vi "Compile UEGO Channels.vi"(8 "error in (no error)":errorcluster, 10 "Name":string, 11 "Device Item Ref in":T6 format="%.0x") -> (0 "error out":errorcluster, 1 "UEGO Engine Data":T2 {"Ordered Channels" format="%.0x"; "RT IDs"."Slot #" max=15; "RT IDs"."Chip Address (A2 A1 A0)" max=7}, 2 "Initial UEGO SPI CMDs":u64[](array[numeric]), 3 "Device Item Ref out":T6 format="%.0x", 5 "RT UEGO Settling Time Data":T1)   [LabVIEW 2014, in "SLSC configuration System Explorer.lvlib"]
uses:
  SLSC configuration System Explorer.lvlib
  <vilib>/NI Veristand/Custom Device API/Custom Device Item Ref.ctl
  Shared/Type Defs/RT Engine Data.ctl
  Shared/Type Defs/RT IDs.ctl
  Shared/SPI Utility/Slot #.ctl
  Shared/MCP23S17/Chip Address.ctl
  Engine/Type Defs/RT UEGO Setting Time Data.ctl
  Shared/UEGO Board/Bank Calibration States.ctl
  Shared/UEGO Board/Calibration State.ctl
  Shared/Constants.vi
  <vilib>/NI Veristand/Custom Device API/Get Item Property (U32).vi
  <vilib>/NI Veristand/Custom Device Tools/Custom Device Utility Library/Custom Device Utility Library.lvlib
  Shared/SLSC configuration Shared.lvlib
  <vilib>/NI Veristand/Custom Device API/Custom Device API.lvlib
  Engine/SLSC configuration Engine.lvlib
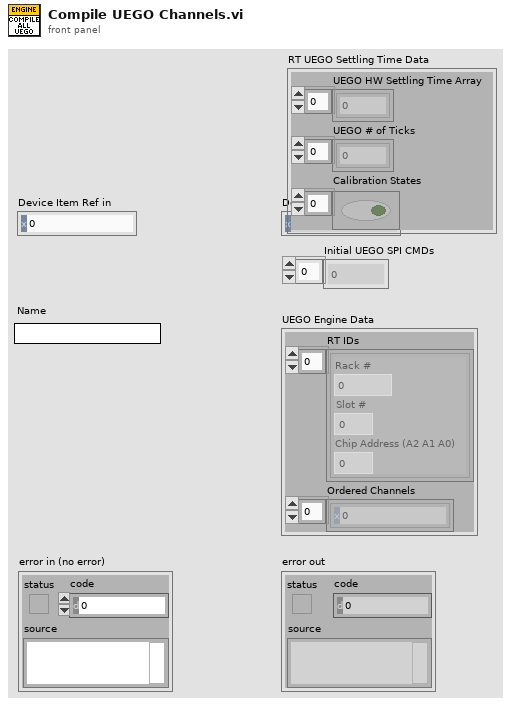
[diagram p1: front panel]
types:
  T1 = typedef "SLSC configuration Engine.lvlib/RT UEGO Setting Time Data.ctl" = cluster{"UEGO HW Settling Time Array":u32[], "UEGO # of Ticks":u32[], "Calibration States":bool[]}
  T2 = typedef "SLSC configuration Shared.lvlib/RT Engine Data.ctl" = cluster{"RT IDs":T3[], "Ordered Channels":T6[]}
  T3 = typedef "SLSC configuration Shared.lvlib/RT IDs.ctl" = cluster{"Rack #":u8, "Slot #":T4, "Chip Address (A2 A1 A0)":T5}
  T4 = typedef "SLSC configuration Shared.lvlib/Slot #.ctl" = u8
  T5 = typedef "SLSC configuration Shared.lvlib/Chip Address.ctl" = u8
  T6 = typedef "Custom Device API.lvlib/Custom Device Item Ref.ctl" = u64
  T7 = typedef "SLSC configuration Shared.lvlib/Bank Calibration States.ctl" = T8[]
  T8 = typedef "SLSC configuration Shared.lvlib/Calibration State.ctl" = bool
  T9 = typedef "SLSC configuration Shared.lvlib/Card Position.ctl" = cluster{"Rack #":u8, "Slot #":T4}
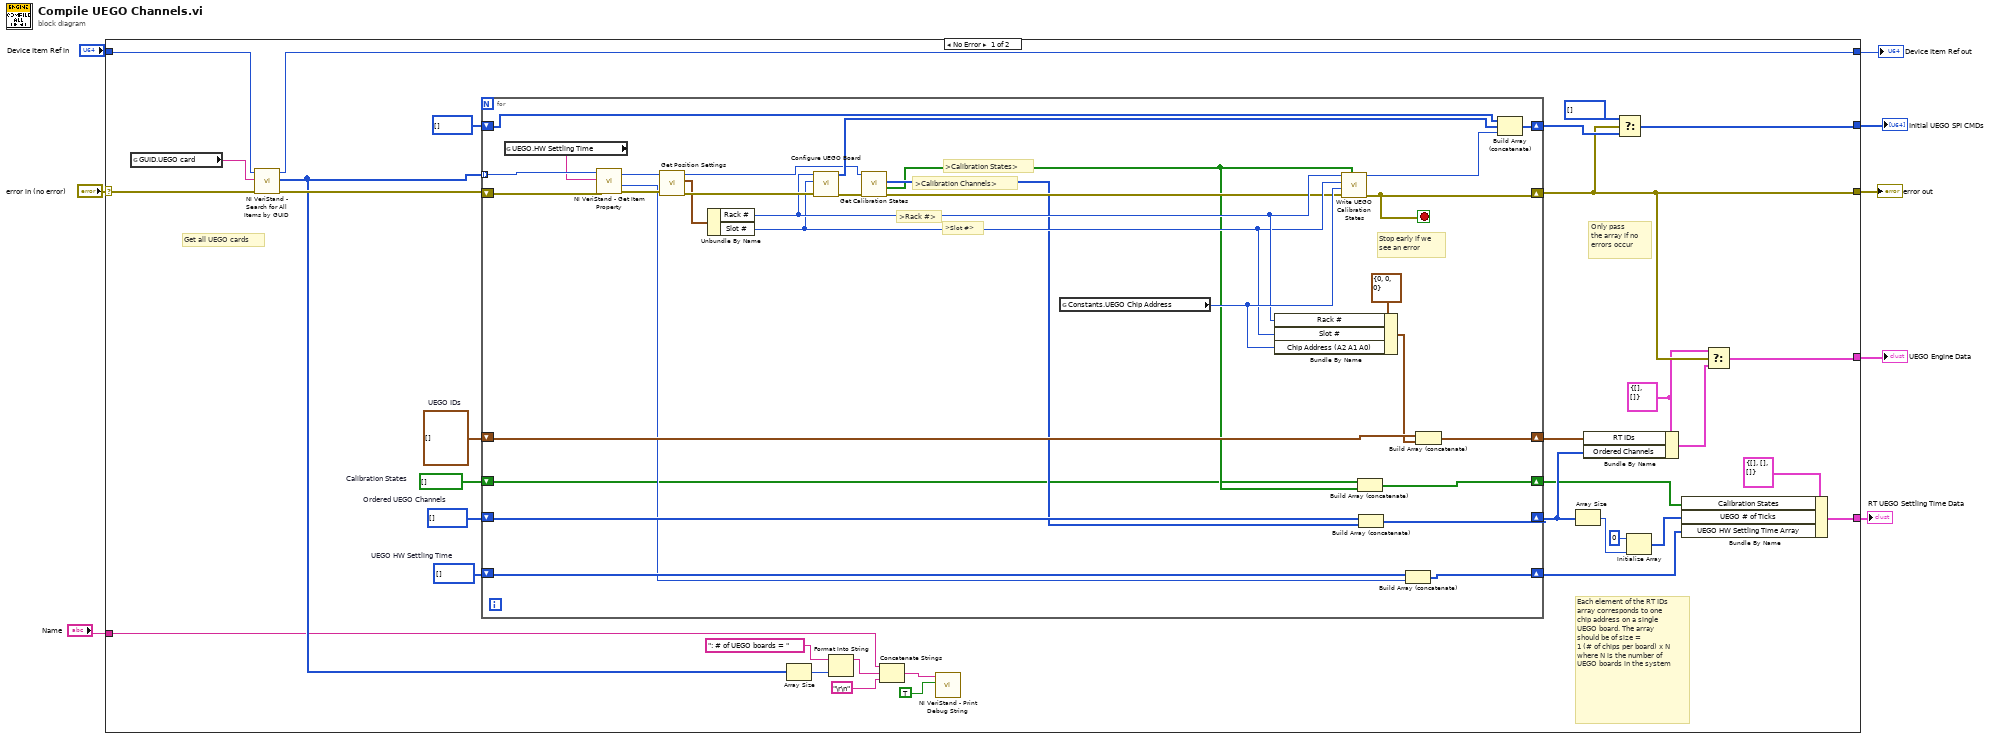
[diagram p0: block diagram]
diagram:
  n1 = case shown="No Error" "error in (no error)" {
    selector: "error in (no error)" -> [w40 w75]
    tunnel: [w30 w75] -> w8
    tunnel: "Device Item Ref in" -> [w35 w74]
    tunnel: [w27 _] -> w5
    tunnel: [w31 _] -> w4
    tunnel: [w34 w74] -> w3
    tunnel: "Name" -> [w19 _]
    tunnel: [w12 _] -> w1
    frame No Error {
      w10 = T7 []  # Calibration States
      w18 = u32[] []  # UEGO HW Settling Time
      w29 = T2 {"RT IDs"=[], "Ordered Channels"=[]} ("FIU Engine Data")
      w37 = T6[] []  # Ordered UEGO Channels
      w38 = T3[] []  # UEGO IDs
      # "Only pass\nthe array if no\nerrors occur"
      # "Get all UEGO cards"
      # "Each element of the RT IDs array corresponds to one chip address on a single UEGO board. The array should be of size =\n1 (# of chips per board) x N where N is the number of UEGO boards in the system"
      n2 = global read "Constants.vi" "GUID.UEGO card"() -> (w42:string)
      n3 = call <vilib>:"NI VeriStand - Search for All Items by GUID.vi"("error in"=w40, "Item GUID"=w42, "Section Ref in"=w35) -> ("error out"=w41:errorcluster, "Item Refs"=w20:T6[], "Section Ref out"=w34:T6)  [unwired: 5 in, 1 out]
      n4 = for {
        tunnel: w20 -> [w53] mode=indexing
        shift-right: [w65] -> w30
        shift-left: w41 -> [w54]
        shift-right: [w70] -> w33
        shift-left: u64[] [] ("SPI FIFO Messages") -> [w73]
        shift-right: [w68] -> w36
        shift-left: w38 -> [w69]
        shift-right: [w66] -> w17
        shift-left: w37 -> [w67]
        shift-right: [w47] -> w13
        shift-left: w18 -> [w48]
        shift-right: [w43] -> w9
        shift-left: w10 -> [w44]
        stop <- w65 stop-if-true
        # ">Calibration States>"
        # "Stop early if we\nsee an error"
        # ">Calibration Channels>"
        # ">Slot #>"
        # ">Rack #>"
        n5 = global read "Constants.vi" "UEGO.HW Settling Time"() -> (w50:string)
        n6 = call-poly <vilib>:"NI VeriStand - Get Item Property.vi"("error in (no error)"=w54, "Property Name"=w50, "Item Ref in"=w53) -> ("error out"=w52:errorcluster, "Value"=w46:u32, "Item Ref out"=w51:T6)  [unwired: 5 in, 1 out]
        n7 = call "Get Position Settings.vi"("error in (no error)"=w52, "Item Ref in"=w51) -> ("error out"=w61:errorcluster, "Card Position"=w60:T9, "Item Ref out"=w56:T6)  [unwired: 7 in]
        n8 = Unbundle By Name(w60) -> ("Rack #"=w59:u8, "Slot #"=w58:T4)
        n9 = call "Configure UEGO Board.vi"("error in (no error)"=w61, "Slot #"=w58, "Rack #"=w59) -> ("error out"=w57:errorcluster, "SPI FIFO Messages"=w72:u64[])  [unwired: 7 in]
        n10 = call "Get Calibration States.vi"("error in (no error)"=w57, "Item Ref in"=w56) -> ("error out"=w55:errorcluster, "UEGO Calibration States"=w45:T7, "Ordered UEGO Channels"=w49:T6[])  [unwired: 6 in, 1 out]
        n11 = global read "Constants.vi" "Constants.UEGO Chip Address"() -> (w64:u8)
        n12 = Bundle By Name(cluster=T3 {"Rack #"=0, "Slot #"=0, "Chip Address (A2 A1 A0)"=0}, "Rack #"=w59, "Slot #"=w58, "Chip Address (A2 A1 A0)"=w64) -> (w62:T3)
        n13 = call "Write UEGO Calibration States.vi"("UEGO Calibration States"=w45, "error in (no error)"=w55, "Chip Address (A2 A1 A0)"=w64, "Slot #"=w58, "Rack #"=w59) -> ("error out"=w65:errorcluster, "FIFO SPI Message"=w71:u64)  [unwired: 4 in, 1 out]
        n14 = Build Array (concatenate)(w44, w45) -> (w43:T7)
        n15 = Build Array (concatenate)(w67, w49) -> (w66:T6[])
        n16 = Build Array (concatenate)(w48, w46) -> (w47:u32[])
        n17 = Build Array (concatenate)(w69, w62) -> (w68:T3[])
        n18 = Build Array (concatenate)(w73, w72, w71) -> (w70:u64[])
      }
      n19 = Array Size(array=w20) -> (size(s)=w25:i32)
      n20 = Format Into String(initial string=": # of UEGO boards = ", w25) -> (resulting string=w22:string)  [unwired: 2 in, 1 out]
      n21 = Concatenate Strings(w19, w22, "\r\n") -> (w23:string)
      n22 = call <vilib>:"NI VeriStand - Print Debug String.vi"("Add to log file? (T)"=TRUE, "Message"=w23) -> ()  [unwired: 9 in, 1 out]
      n23 = Array Size(array=w17) -> (size(s)=w11:i32)
      n24 = Bundle By Name(cluster=w29, "RT IDs"=w36, "Ordered Channels"=w17) -> (w28:T2)
      n25 = Select(t=u64[] [], s=w30, f=w33) -> (s? t:f=w31:u64[])
      n26 = Initialize Array(u32 0 ("Value"), w11) -> (w14:u32[])
      n27 = Bundle By Name(cluster=T1 {"UEGO HW Settling Time Array"=[], "UEGO # of Ticks"=[], "Calibration States"=[]}, "Calibration States"=w9, "UEGO # of Ticks"=w14, "UEGO HW Settling Time Array"=w13) -> (w12:T1)
      n28 = Select(t=w29, s=w30, f=w28) -> (s? t:f=w27:T2)
    }
    frame Error {
    }
  }
  "error out" <- w8
  "Device Item Ref out" <- w3
  "UEGO Engine Data" <- w5
  "Initial UEGO SPI CMDs" <- w4
  "RT UEGO Settling Time Data" <- w1
